vi "7-1.vi"() -> ()   [LabVIEW 2022 SP3, in "AoC22.lvlib"]
uses:
  AoC22.lvlib
  Disk Node.ctl
  <vilib>/IlluminatedG/lv-stream/Stream.lvlib
panel:
  out "Numeric":u64
  out "ABORT":bool
  in  "milliseconds to wait":u32
  out "elements":i32[](array[numeric])
  out "Array":T1[](array[typedef])
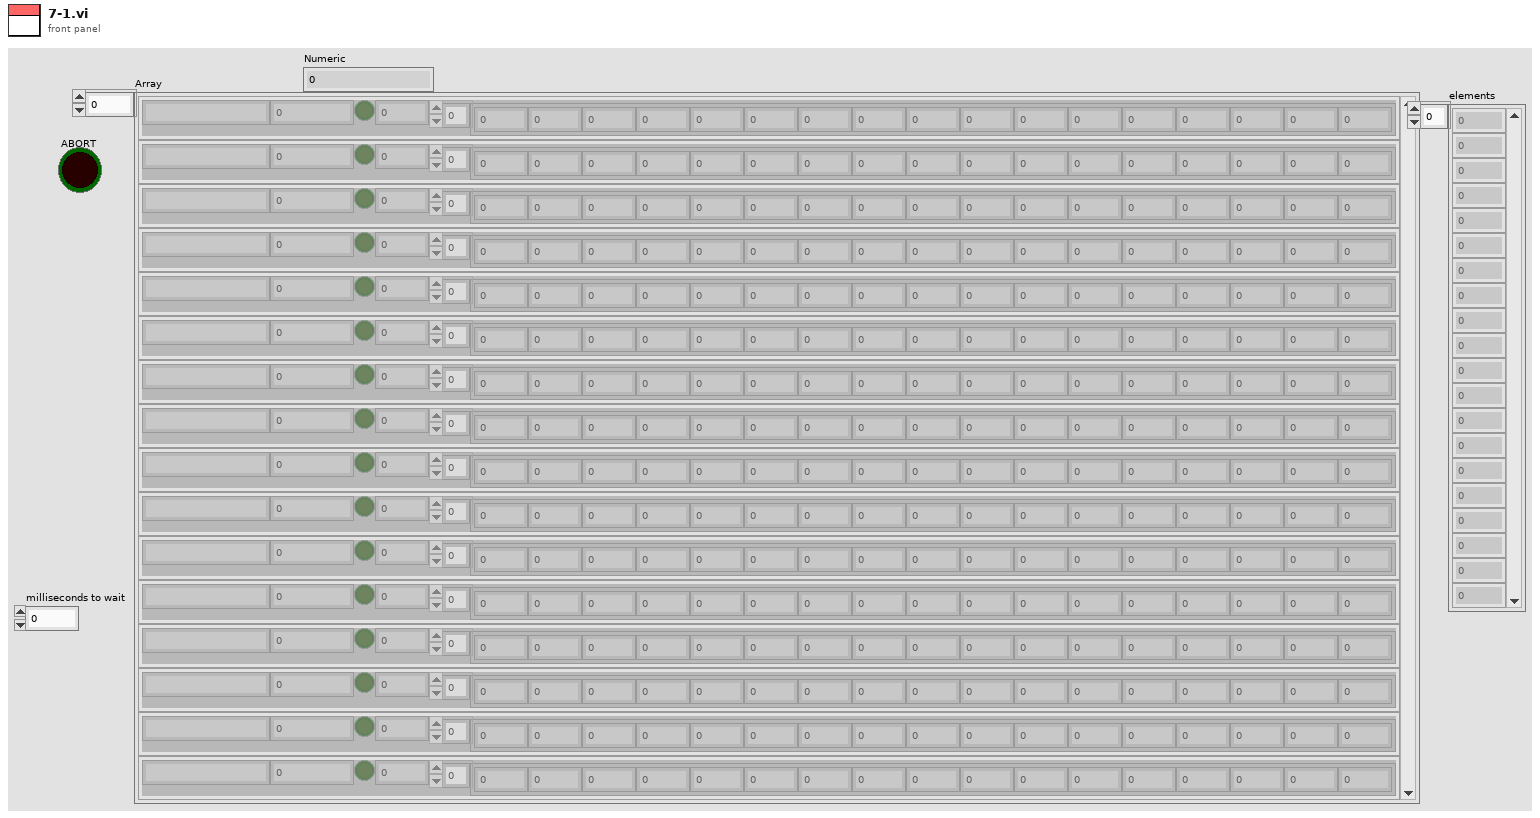
[diagram p1: front panel]
types:
  T1 = typedef "AoC22.lvlib/Disk Node.ctl" = cluster{"Name":string, "Size":u32, "Directory":bool, "Parent":i32, "Children":i32[]}
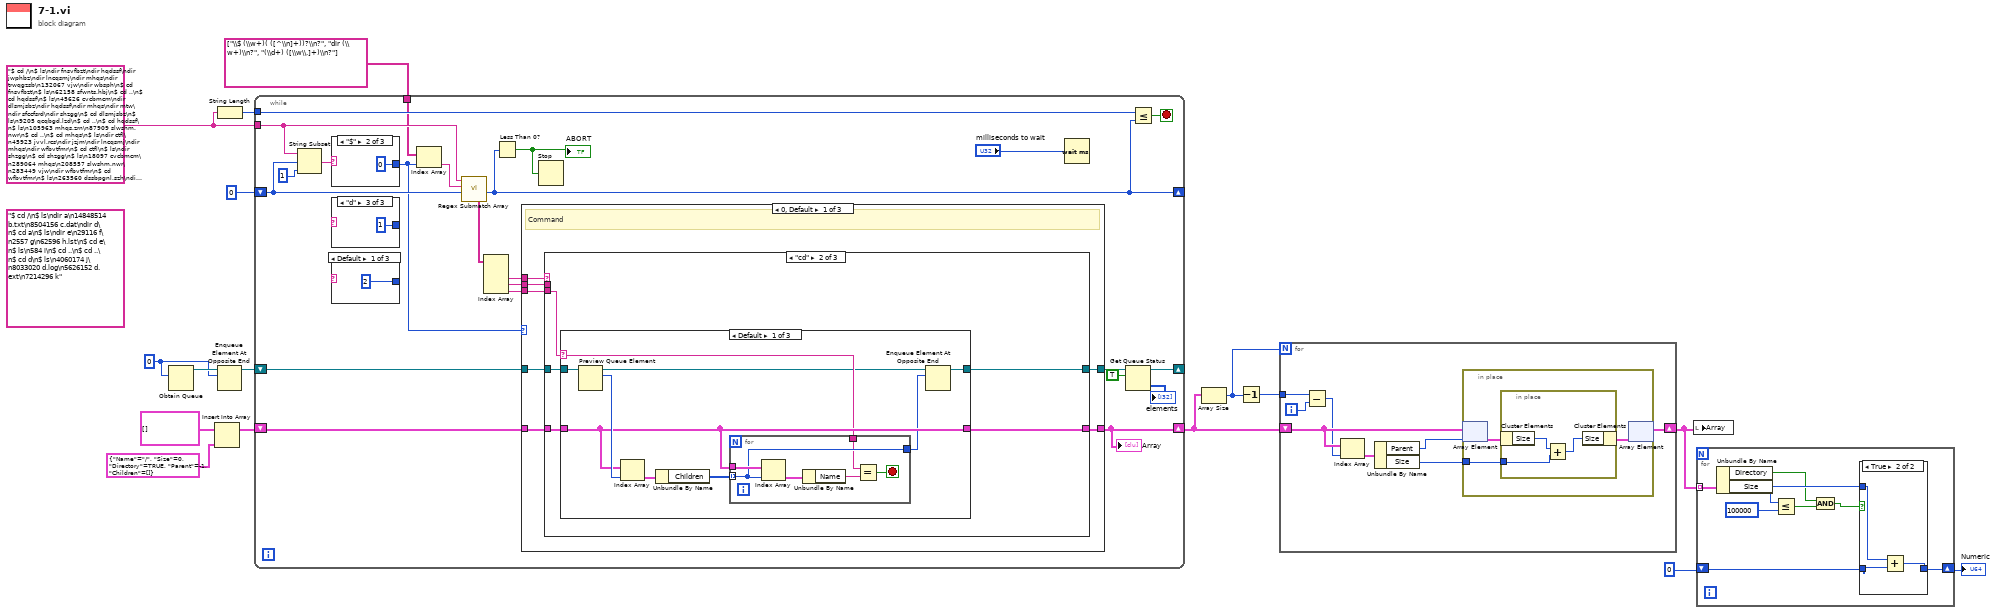
[diagram p0: block diagram]
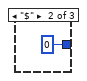
[diagram p3: hidden frame]
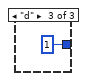
[diagram p4: hidden frame]
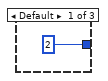
[diagram p5: hidden frame]
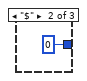
[diagram p6: hidden frame]
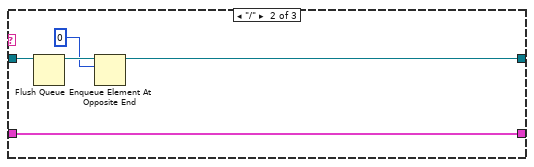
[diagram p8: hidden frame]
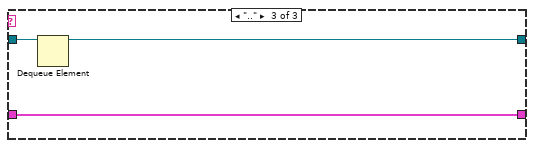
[diagram p9: hidden frame]
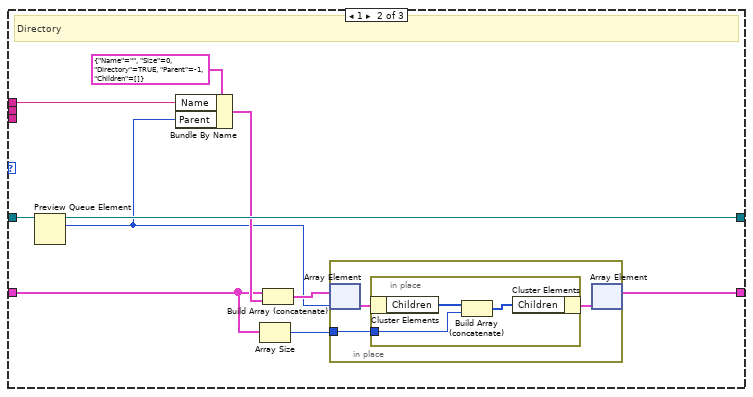
[diagram p11: hidden frame]
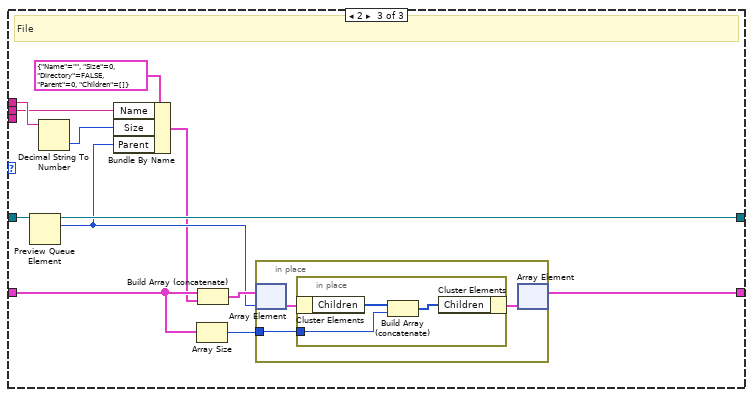
[diagram p12: hidden frame]
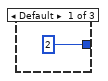
[diagram p13: hidden frame]
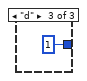
[diagram p14: hidden frame]
diagram:
  (unwired) "$ cd /\n$ ls\ndir a\n14848514 b.txt\n8504156 c.dat\ndir d\n$ cd a\n$ ls\ndir e\n29116 f\n2557 g\n62596 h.lst\n$ cd e\n$ ls\n584 i\n$ cd ..\n$ cd ..\n$ cd d\n$ ls\n4060174 j\n8033020 d.log\n5626152 d.ext\n7214296 k"
  w8 = 0
  w1 = "$ cd /\n$ ls\ndir fnsvfbzt\ndir hqdssf\ndir jwphbz\ndir lncqsmj\ndir mhqs\ndir trwqgzsb\n132067 vjw\ndir wbsph\n$ cd fnsvfbzt\n$ ls\n62158 sfwnts.hbj\n$ cd ..\n$ cd hqdssf\n$ ls\n45626 cvcbmcm\ndir dlsmjsbz\ndir hqdssf\ndir mhqs\ndir mtw\ndir sfccfsrd\ndir shzgg\n$ cd dlsmjsbz\n$ ls\n9205 qcqbgd.lzd\n$ cd ..\n$ cd hqdssf\n$ ls\n105963 mhqs.zrn\n87909 slwshm.nwr\n$ cd ..\n$ cd mhqs\n$ ls\ndir ctfl\n45923 jvvl.rcs\ndir jzjm\ndir lncqsmj\ndir mhqs\ndir wfbvtfmr\n$ cd ctfl\n$ ls\ndir shzgg\n$ cd shzgg\n$ ls\n18097 cvcbmcm\n289064 mhqs\n208557 slwshm.nwr\n283449 vjw\ndir wfbvtfmr\n$ cd wfbvtfmr\n$ ls\n263560 dssbpgnl.szh\ndir hnqjmq\n76551 jvvl.rcs\n195911 lncqsmj\n185776 slwshm.nwr\n$ cd hnqjmq\n$ ls\n3307 rjd.lgh\n$ cd ..\n$ cd ..\n$ cd ..\n$ cd ..\n$ cd jzjm\n$ ls\n31719 rjjrg.pjq\n$ cd ..\n$ cd lncqsmj\n$ ls\ndir mhqs\n$ cd mhqs\n$ ls\n138296 wfbvtfmr\n$ cd ..\n$ cd ..\n$ cd mhqs\n$ ls\n175499 jvvl.rcs\ndir rqznrr\n108476 slwshm.nwr\n199853 vjw\n$ cd rqznrr\n$ ls\n105075 shslmlt.spg\n$ cd ..\n$ cd ..\n$ cd wfbvtfmr\n$ ls\n131522 rjjrg.pjq\n$ cd ..\n$ cd ..\n$ cd mtw\n$ ls\ndir dcgpfrsf\ndir gwqm\n188911 hqdssf\n34693 jvvl.rcs\ndir shzgg\n$ cd dcgpfrsf\n$ ls\n47863 dfwthflp.jwq\n203815 dqbqbps.prq\ndir mhqs\n183653 rqjqpm.bbr\n220694 vjw\n$ cd mhqs\n$ ls\n74450 tjpn\n$ cd ..\n$ cd ..\n$ cd gwqm\n$ ls\ndir trghjhvs\n$ cd trghjhvs\n$ ls\ndir shzgg\n2620 slwshm.nwr\n$ cd shzgg\n$ ls\n73435 shzgg.bbf\n$ cd ..\n$ cd ..\n$ cd ..\n$ cd shzgg\n$ ls\n184378 rjjrg.pjq\n$ cd ..\n$ cd ..\n$ cd sfccfsrd\n$ ls\n87317 ccvs.phq\ndir cqmgf\ndir cssmfv\ndir hhhqdmz\n17971 mhqs\ndir mvjttqr\n264394 slwshm.nwr\ndir stdzptb\ndir tcddd\ndir zmrt\ndir zqqtb\n$ cd cqmgf\n$ ls\n202804 tcrqqlgs\n$ cd ..\n$ cd cssmfv\n$ ls\n13440 jnhzrtfd\n$ cd ..\n$ cd hhhqdmz\n$ ls\ndir fdbpld\n272827 jftd.lml\ndir prqbhbv\ndir wbzvmz\n$ cd fdbpld\n$ ls\ndir bgrnz\ndir dcdj\n78284 jqqfc.tzz\n147731 lbdsh.plp\n269235 ntf.gmq\n$ cd bgrnz\n$ ls\ndir qzs\ndir rcv\ndir wmrmhdd\n$ cd qzs\n$ ls\n156779 lncqsmj.gnf\n$ cd ..\n$ cd rcv\n$ ls\n224927 dvbw.svf\ndir hqdssf\ndir jjmsqft\n255189 mhqs.pcl\ndir mvgqtlm\ndir pjs\ndir sljw\n$ cd hqdssf\n$ ls\n63099 blpdwd\n96035 jvvl.rcs\n40533 lvpsmzw\n205031 rjjrg.pjq\n59874 shzgg.ldg\ndir zdnfpwlw\n$ cd zdnfpwlw\n$ ls\n109325 hqdssf.fmj\n41775 jfqhq.tdn\n203744 nprghch.zjb\ndir qfs\ndir rzctqrgm\ndir shzgg\n$ cd qfs\n$ ls\n234449 vjw\n$ cd ..\n$ cd rzctqrgm\n$ ls\n99041 cvcbmcm\n$ cd ..\n$ cd shzgg\n$ ls\n149752 mhqs.bds\n126331 rjjrg.pjq\n75464 vbcjqdjv\n$ cd ..\n$ cd ..\n$ cd ..\n$ cd jjmsqft\n$ ls\n47522 shzgg\n$ cd ..\n$ cd mvgqtlm\n$ ls\ndir tgtbj\ndir tmrsn\ndir vpv\n$ cd tgtbj\n$ ls\n86585 lbmv.jcr\n202755 rjjrg.pjq\n$ cd ..\n$ cd tmrsn\n$ ls\n150980 hqdssf.hmh\n$ cd ..\n$ cd vpv\n$ ls\n197783 jvvl.rcs\n$ cd ..\n$ cd ..\n$ cd pjs\n$ ls\n216539 cvcbmcm\n159509 jgfphj\n195297 pdgnb.qjd\n162974 rjjrg.pjq\n$ cd ..\n$ cd sljw\n$ ls\n61689 hqdssf.bbn\n$ cd ..\n$ cd ..\n$ cd wmrmhdd\n$ ls\n92888 msgcqfbf\n$ cd ..\n$ cd ..\n$ cd dcdj\n$ ls\n99280 mclcnw\n$ cd ..\n$ cd ..\n$ cd prqbhbv\n$ ls\n102589 bqlcds.pqp\n107625 mhqs\n281871 mvwvdtd.dzf\n$ cd ..\n$ cd wbzvmz\n$ ls\n287371 tnwgfw\n$ cd ..\n$ cd ..\n$ cd mvjttqr\n$ ls\ndir dtf\ndir frcqdb\ndir hqdssf\n55645 slwshm.nwr\ndir zdzchmtq\n$ cd dtf\n$ ls\n121764 cvcbmcm\n279094 lncqsmj\n68484 slwshm.nwr\n278387 vjw\n$ cd ..\n$ cd frcqdb\n$ ls\n233216 lncqsmj.mbd\n217901 slwshm.nwr\n$ cd ..\n$ cd hqdssf\n$ ls\ndir dgdtm\n260973 qnt\n231311 thdrddd.zmj\n160399 vjw\ndir vpqjmmf\n197241 vqvzsv.nzg\n$ cd dgdtm\n$ ls\ndir cnshbf\n173312 vjw\n$ cd cnshbf\n$ ls\n72788 hqdssf.mhc\n122945 rjjrg.pjq\n$ cd ..\n$ cd ..\n$ cd vpqjmmf\n$ ls\n127969 hqdssf.stc\n267724 lncqsmj\n55890 mhqs.mql\ndir tsbtz\n$ cd tsbtz\n$ ls\n244065 qqfnbd.nqv\n59649 qttbcgd.vtj\n$ cd ..\n$ cd ..\n$ cd ..\n$ cd zdzchmtq\n$ ls\n271886 lmphsmv\ndir nncghrr\n$ cd nncghrr\n$ ls\n180468 rjjrg.pjq\n$ cd ..\n$ cd ..\n$ cd ..\n$ cd stdzptb\n$ ls\n19398 frsztqqz.mnc\n$ cd ..\n$ cd tcddd\n$ ls\ndir hqdssf\n71084 jvvl.rcs\ndir wnzhld\n$ cd hqdssf\n$ ls\n178907 gcslqrn\n$ cd ..\n$ cd wnzhld\n$ ls\n206073 hpdnj\n$ cd ..\n$ cd ..\n$ cd zmrt\n$ ls\ndir bmfgjr\ndir bpztq\ndir chsh\ndir dpjhn\n288144 mhqs.zvb\n$ cd bmfgjr\n$ ls\n189592 jhmgm\n$ cd ..\n$ cd bpztq\n$ ls\n184906 rjjrg.pjq\n$ cd ..\n$ cd chsh\n$ ls\n110753 jvvl.rcs\ndir lncqsmj\ndir njdgplj\ndir qhpplfnd\n190460 rjjrg.pjq\n144668 wfbvtfmr.flv\n$ cd lncqsmj\n$ ls\ndir pzd\n$ cd pzd\n$ ls\n287833 vhfjdg.jrz\n$ cd ..\n$ cd ..\n$ cd njdgplj\n$ ls\ndir cbvz\ndir vfhj\n$ cd cbvz\n$ ls\ndir rtpcsrf\n$ cd rtpcsrf\n$ ls\n240018 wfbvtfmr\n$ cd ..\n$ cd ..\n$ cd vfhj\n$ ls\n152840 cbbrgc.wnq\n243656 hqdssf\n36325 hqdssf.fhn\n$ cd ..\n$ cd ..\n$ cd qhpplfnd\n$ ls\n206490 dfththnq.vnm\n$ cd ..\n$ cd ..\n$ cd dpjhn\n$ ls\n127322 rjjrg.pjq\ndir shzgg\n$ cd shzgg\n$ ls\n165774 cvcbmcm\n$ cd ..\n$ cd ..\n$ cd ..\n$ cd zqqtb\n$ ls\ndir ljnmbqvd\n60485 pcz.snl\n274930 slwshm.nwr\n131928 vqm\n51341 wfbvtfmr.stc\n$ cd ljnmbqvd\n$ ls\n268048 bdbjn\ndir fjh\ndir qpclpbz\ndir rqpljw\ndir tzjftf\n255809 vjw\n243604 wfbvtfmr.rzb\n$ cd fjh\n$ ls\n180021 hqdssf.rqs\n$ cd ..\n$ cd qpclpbz\n$ ls\n109952 blmm.nsv\ndir dltbt\ndir htbzp\n287761 mfbd\ndir mhqs\ndir vgbvrwvn\ndir wmhd\n$ cd dltbt\n$ ls\n205121 dfzlcv.hjf\n56409 hpqhhmb.sss\n233277 hqdssf.qcb\n187838 mbmcfhf.fnj\ndir rrqjn\ndir swrgj\n151306 tqjzq.dmg\n$ cd rrqjn\n$ ls\n240447 lncqsmj\n$ cd ..\n$ cd swrgj\n$ ls\ndir lnnwdbt\ndir sgjsn\ndir wfbvtfmr\n$ cd lnnwdbt\n$ ls\n213111 tnn.bhq\n$ cd ..\n$ cd sgjsn\n$ ls\ndir wpprqhs\n$ cd wpprqhs\n$ ls\ndir hqdssf\n$ cd hqdssf\n$ ls\n209286 qbdfzdzw.sgp\n$ cd ..\n$ cd ..\n$ cd ..\n$ cd wfbvtfmr\n$ ls\n199298 hqdssf.chs\n123953 rjjrg.pjq\n$ cd ..\n$ cd ..\n$ cd ..\n$ cd htbzp\n$ ls\ndir bmfr\n68162 bzwcswr.mlv\n284074 dtzwf\n270421 jpsvh.ncc\ndir mwbvz\n95631 shzgg.tbf\n44434 vjw\n$ cd bmfr\n$ ls\n19937 shzgg\n$ cd ..\n$ cd mwbvz\n$ ls\n156668 rjjrg.pjq\n$ cd ..\n$ cd ..\n$ cd mhqs\n$ ls\n111821 ftrv.zcw\ndir jsnlcn\ndir mhqs\ndir rjdwmb\ndir sfmrwgd\n$ cd jsnlcn\n$ ls\n7527 smqts.cnc\ndir svdw\n$ cd svdw\n$ ls\n173846 vjtrp\n$ cd ..\n$ cd ..\n$ cd mhqs\n$ ls\ndir hswdjgg\n30326 rjjrg.pjq\n$ cd hswdjgg\n$ ls\n285037 jvvl.rcs\n$ cd ..\n$ cd ..\n$ cd rjdwmb\n$ ls\n219498 twl.lmw\n$ cd ..\n$ cd sfmrwgd\n$ ls\n168290 ltwpm.fjl\n$ cd ..\n$ cd ..\n$ cd vgbvrwvn\n$ ls\ndir bswv\ndir hqdssf\ndir mhqs\n$ cd bswv\n$ ls\n121032 cncdt\ndir jrbmlg\ndir lncqsmj\ndir mhmgn\n65380 rjjrg.pjq\ndir wfbvtfmr\n$ cd jrbmlg\n$ ls\n37975 shzgg.bnq\n$ cd ..\n$ cd lncqsmj\n$ ls\n114558 jvvl.rcs\ndir mhqs\ndir nfn\ndir nhlbfq\n141816 phtt.phj\n181530 vjw\n224510 zmzp.jwg\n$ cd mhqs\n$ ls\ndir wpnw\n$ cd wpnw\n$ ls\n286077 lncqsmj.cld\n$ cd ..\n$ cd ..\n$ cd nfn\n$ ls\n269740 cvcbmcm\n87123 mhqs.nst\n61029 mhqs.vhb\n211712 slwshm.nwr\n$ cd ..\n$ cd nhlbfq\n$ ls\n247458 lncqsmj\n$ cd ..\n$ cd ..\n$ cd mhmgn\n$ ls\n85806 vjw\n$ cd ..\n$ cd wfbvtfmr\n$ ls\n275888 cvvhvg.pwv\n151703 gnbm\n61419 grcfbwdp\n150382 gzdmzj.wpc\ndir mtrqcwrd\n112827 nbtjlnt.srg\n$ cd mtrqcwrd\n$ ls\n273564 shzgg.tbm\n$ cd ..\n$ cd ..\n$ cd ..\n$ cd hqdssf\n$ ls\n72227 ccvwdrs.dsf\n141028 dctbz.spr\ndir shzgg\n277461 slwshm.nwr\n94390 stgp.trm\n24297 vgdzsrrl.dhg\n$ cd shzgg\n$ ls\n143437 lncqsmj.vpl\n78418 pbdwbmtd.nlp\n28173 vlfj.tps\n$ cd ..\n$ cd ..\n$ cd mhqs\n$ ls\n97312 jvvl.rcs\ndir qqfbsz\n42472 rjjrg.pjq\ndir wfbvtfmr\n$ cd qqfbsz\n$ ls\ndir lncqsmj\ndir mhqs\n$ cd lncqsmj\n$ ls\n186873 wfbvtfmr.lfh\n$ cd ..\n$ cd mhqs\n$ ls\ndir wfbvtfmr\n$ cd wfbvtfmr\n$ ls\n234441 gsjwsn\n$ cd ..\n$ cd ..\n$ cd ..\n$ cd wfbvtfmr\n$ ls\n55214 dgf\ndir fdtz\n6756 jvvl.rcs\n226995 rpsjvr.wpb\n68993 vjw\n$ cd fdtz\n$ ls\ndir rdzsjm\n$ cd rdzsjm\n$ ls\ndir mjgfpvc\n$ cd mjgfpvc\n$ ls\ndir vfcq\n$ cd vfcq\n$ ls\ndir fmtfm\n$ cd fmtfm\n$ ls\n200137 dvbqjq\n$ cd ..\n$ cd ..\n$ cd ..\n$ cd ..\n$ cd ..\n$ cd ..\n$ cd ..\n$ cd ..\n$ cd wmhd\n$ ls\ndir hnn\ndir rzt\n$ cd hnn\n$ ls\n16335 wfbvtfmr.vhw\n262909 zgtln.dwc\n$ cd ..\n$ cd rzt\n$ ls\n285086 mhqs.vsg\ndir qnr\n$ cd qnr\n$ ls\n290611 llnp.hsh\n$ cd ..\n$ cd ..\n$ cd ..\n$ cd ..\n$ cd rqpljw\n$ ls\n267152 jbv\n$ cd ..\n$ cd tzjftf\n$ ls\n258707 cnfb.dgv\n17087 hqdssf.dtd\n92075 nwvtww\ndir qblrnn\ndir tdg\n$ cd qblrnn\n$ ls\ndir brrqp\ndir frqcc\n25504 jvvl.rcs\ndir lncqsmj\ndir mhqs\n107908 rjjrg.pjq\n286918 rngbhp.ntg\ndir shzgg\ndir wcnh\ndir wfbvtfmr\n$ cd brrqp\n$ ls\n270783 wfbvtfmr\n$ cd ..\n$ cd frqcc\n$ ls\ndir clj\n7502 lncqsmj\ndir mnsbr\n73859 scwltjwh.cqd\n29920 vjw\ndir wpplgrc\n$ cd clj\n$ ls\n31407 grm.pwv\n$ cd ..\n$ cd mnsbr\n$ ls\ndir wfbvtfmr\n99467 whsrtf.gff\n$ cd wfbvtfmr\n$ ls\n81283 cvcbmcm\n$ cd ..\n$ cd ..\n$ cd wpplgrc\n$ ls\n285496 lncqsmj.hwq\n$ cd ..\n$ cd ..\n$ cd lncqsmj\n$ ls\n8972 jvvl.rcs\n$ cd ..\n$ cd mhqs\n$ ls\n119520 hqdssf.tbn\n$ cd ..\n$ cd shzgg\n$ ls\n180825 lncqsmj.rsg\n23507 wfbvtfmr\n$ cd ..\n$ cd wcnh\n$ ls\n98662 tmwrh\n220468 wml.sht\n$ cd ..\n$ cd wfbvtfmr\n$ ls\n283178 hqdssf.ctf\n$ cd ..\n$ cd ..\n$ cd tdg\n$ ls\n283636 cvcbmcm\n117742 gsqzjfn.pmp\n176660 lncqsmj\ndir pbdgbsts\ndir znvv\n$ cd pbdgbsts\n$ ls\n92092 vjw\n$ cd ..\n$ cd znvv\n$ ls\n41213 hqdssf.rnn\ndir pcttrtd\n$ cd pcttrtd\n$ ls\n16759 mhqs.gpb\n$ cd ..\n$ cd ..\n$ cd ..\n$ cd ..\n$ cd ..\n$ cd ..\n$ cd ..\n$ cd shzgg\n$ ls\n19544 bcn.rws\ndir fqwpwcq\ndir hngpzst\ndir hqdssf\ndir shzgg\ndir vgjr\ndir wfbvtfmr\n$ cd fqwpwcq\n$ ls\n269576 mhqs\ndir pmfv\n$ cd pmfv\n$ ls\n175725 jvvl.rcs\n29161 pnbm.mlr\n$ cd ..\n$ cd ..\n$ cd hngpzst\n$ ls\n18430 cvcbmcm\ndir fgzlgbm\ndir hqdssf\n378 rjjrg.pjq\ndir zjlnsztt\n$ cd fgzlgbm\n$ ls\n134751 dwlfbfjp\ndir hqdssf\n227313 jvvl.rcs\ndir lncqsmj\ndir mhqs\ndir qfjmtvpv\ndir qzm\n114934 shzgg.jdf\n187091 zpgbdnl.twq\n$ cd hqdssf\n$ ls\n87131 bdmdpdf.cqg\ndir fdc\ndir gwgp\n$ cd fdc\n$ ls\n116738 cvcbmcm\n$ cd ..\n$ cd gwgp\n$ ls\ndir qdvss\ndir rpwzw\ndir wfbvtfmr\n$ cd qdvss\n$ ls\n111546 wqnsrnh\n$ cd ..\n$ cd rpwzw\n$ ls\n183614 lfjqvff\n129803 rdwd\n$ cd ..\n$ cd wfbvtfmr\n$ ls\n266779 mhqs\n189793 slwshm.nwr\n279894 sncqtvwp.mff\n40520 vjw\n$ cd ..\n$ cd ..\n$ cd ..\n$ cd lncqsmj\n$ ls\n257714 dtcjv.lsd\n69877 shzgg\n267645 vjw\n$ cd ..\n$ cd mhqs\n$ ls\n257031 stsfrb.gvs\n$ cd ..\n$ cd qfjmtvpv\n$ ls\ndir mhqs\n$ cd mhqs\n$ ls\n91378 wldhvhl\n$ cd ..\n$ cd ..\n$ cd qzm\n$ ls\ndir shn\n$ cd shn\n$ ls\ndir jmmlsvdg\n$ cd jmmlsvdg\n$ ls\n41383 rnlgl.vjv\n$ cd ..\n$ cd ..\n$ cd ..\n$ cd ..\n$ cd hqdssf\n$ ls\ndir mzj\n$ cd mzj\n$ ls\n169639 sgdn\n$ cd ..\n$ cd ..\n$ cd zjlnsztt\n$ ls\n78315 jfj.sgg\n$ cd ..\n$ cd ..\n$ cd hqdssf\n$ ls\n906 rjjrg.pjq\n$ cd ..\n$ cd shzgg\n$ ls\n163015 mhqs.cnb\n$ cd ..\n$ cd vgjr\n$ ls\n129546 hclg.vbl\n286437 hqdssf\ndir lncqsmj\n1552 nhgwff\n279693 qmpdlw\n83645 slwshm.nwr\n$ cd lncqsmj\n$ ls\n233355 fhpjbpjl.tbh\n$ cd ..\n$ cd ..\n$ cd wfbvtfmr\n$ ls\n218452 jvvl.rcs\n47525 rjjrg.pjq\n109880 tctz.rnd\n$ cd ..\n$ cd ..\n$ cd ..\n$ cd jwphbz\n$ ls\ndir bqbwds\ndir mwnzw\n113414 qgdsgfg.ngj\n141013 qtp\n10795 slwshm.nwr\n$ cd bqbwds\n$ ls\n18049 shzgg\n$ cd ..\n$ cd mwnzw\n$ ls\n169353 dtqlr\ndir hlrgzlph\ndir mhqs\n238527 vjw\n$ cd hlrgzlph\n$ ls\n249097 hqdssf\n86490 pwdmzwb\n$ cd ..\n$ cd mhqs\n$ ls\n176337 rjjrg.pjq\n$ cd ..\n$ cd ..\n$ cd ..\n$ cd lncqsmj\n$ ls\ndir jmsw\ndir mcgm\ndir mpc\n233050 rjjrg.pjq\n30757 shzgg\n250575 slwshm.nwr\n$ cd jmsw\n$ ls\ndir hqdssf\ndir nmsbdqhm\ndir wfbvtfmr\n$ cd hqdssf\n$ ls\n44806 lvzm\n$ cd ..\n$ cd nmsbdqhm\n$ ls\ndir czzp\ndir gcp\ndir gsrnmq\ndir rmngvc\ndir vpfq\ndir vpzvb\ndir wccgblsq\n43981 wfbvtfmr\n$ cd czzp\n$ ls\n95330 slwshm.nwr\n82000 wfbvtfmr\n$ cd ..\n$ cd gcp\n$ ls\n229303 ddsppspd.fcn\n$ cd ..\n$ cd gsrnmq\n$ ls\ndir hrsstlt\ndir rzc\n40890 sfpt\n$ cd hrsstlt\n$ ls\n18477 mnpc.tmh\n$ cd ..\n$ cd rzc\n$ ls\n33078 dmfwf\n149792 wfbvtfmr.jnz\ndir zsnmz\n$ cd zsnmz\n$ ls\ndir gzsnl\n69834 lplszs.rvg\n213489 slwshm.nwr\ndir vrnqh\n$ cd gzsnl\n$ ls\n109060 jvvl.rcs\n122307 svtppnvt.wrz\n$ cd ..\n$ cd vrnqh\n$ ls\n94389 jvvl.rcs\n$ cd ..\n$ cd ..\n$ cd ..\n$ cd ..\n$ cd rmngvc\n$ ls\ndir jljbrrgg\n$ cd jljbrrgg\n$ ls\n128554 cvcbmcm\n$ cd ..\n$ cd ..\n$ cd vpfq\n$ ls\n73628 rjjrg.pjq\n$ cd ..\n$ cd vpzvb\n$ ls\n265609 rjjrg.pjq\n$ cd ..\n$ cd wccgblsq\n$ ls\n110134 hffzwm.zfr\n$ cd ..\n$ cd ..\n$ cd wfbvtfmr\n$ ls\n209356 jvvl.rcs\n286105 mtsb.bwd\n234687 vcgnlc.cft\n$ cd ..\n$ cd ..\n$ cd mcgm\n$ ls\n203407 cvcbmcm\n$ cd ..\n$ cd mpc\n$ ls\ndir shzgg\n$ cd shzgg\n$ ls\ndir bnb\n$ cd bnb\n$ ls\n232449 lncqsmj.czs\n$ cd ..\n$ cd ..\n$ cd ..\n$ cd ..\n$ cd mhqs\n$ ls\n116955 jvvl.rcs\n$ cd ..\n$ cd trwqgzsb\n$ ls\n88439 jgphdrnq\n$ cd ..\n$ cd wbsph\n$ ls\ndir mhqs\ndir vgh\n$ cd mhqs\n$ ls\n133965 rfh.zdb\n$ cd ..\n$ cd vgh\n$ ls\n36092 rjjrg.pjq"
  n1 = Obtain Queue(element data type=w8) -> (queue out=w10:refnum<queue>)  [unwired: 4 in, 2 out]
  n2 = Insert Into Array(array=T1[] [], new element=T1 {"Name"="/", "Size"=0, "Directory"=TRUE, "Parent"=-1, "Children"=[]} ("new element/subarray")) -> (w12:T1[])  [unwired: 1 in]
  n3 = Enqueue Element At Opposite End(queue=w10, element=w8) -> (queue out=w9:refnum<queue>)  [unwired: 2 in, 2 out]
  n4 = String Length(string=w1) -> (length=w15:i32)
  n5 = while {
    tunnel: w1 -> [w36]
    shift-right: [w26] -> _
    shift-left: 0 -> [w35]
    tunnel: w15 -> [w39]
    shift-right: [w24] -> _
    shift-left: w9 -> [w18]
    shift-right: [w19] -> w7
    shift-left: w12 -> [w17]
    tunnel: string[] ["\\$ (\\w+)( ([^\\n]+))?\\n?", "dir (\\w+)\\n?", "(\\d+) ([\\w\\.]+)\\n?"] -> [w32]
    stop <- w38 stop-if-true
    n6 = String Subset(string=w36, offset (0)=w35, length (rest)=1 ("length (rest)")) -> (substring=w33:string)
    n7 = case shown="\"$\"" w33 {
      tunnel: [2 0 1] -> w30
      frame Default {
      }
      frame "$" {
      }
      frame "d" {
      }
    }
    n8 = case shown="\"d\"" {
      selector: _ -> [_ _ _]
      tunnel: [2 0 1] -> _
      frame Default {
      }
      frame "$" {
      }
      frame "d" {
      }
    }
    n9 = case shown="Default" {
      selector: _ -> [_ _ _]
      tunnel: [2 0 1] -> _
      frame Default {
      }
      frame "$" {
      }
      frame "d" {
      }
    }
    n10 = Index Array(array=w32, index=w30) -> (element=w31:string)
    n11 = call <vilib>:"Regex Submatch Array.vi"("offset (0)"=w35, "regular expression"=w31, "string"=w36) -> ("offset past match"=w26:i32, "matches"=w37:string[])  [unwired: 6 in, 1 out]
    n12 = Index Array(array=w37) -> (element #2=w29:string, element #3=w28:string, element #4=w20:string)  [unwired: 4 in, 1 out]
    n13 = Less Than 0?(x=w26) -> (x < 0?=w25:bool)
    "ABORT" <- w25
    n14 = case shown="0, Default" w30 {
      tunnel: w29 -> [w52 w91 w112]
      tunnel: w28 -> [w47 _ w111]
      tunnel: w18 -> [w51 w94 w109]
      tunnel: w17 -> [w49 w89 w107]
      tunnel: [w50 w93 w108] -> w27
      tunnel: [w48 w85 w103] -> w19
      tunnel: w20 -> [w46 _ _]
      frame 0, Default {
        # "Command"
        n15 = case shown="\"cd\"" w52 {
          tunnel: w51 -> [w54 w59 w84]
          tunnel: [w54 w57 w84] -> w50
          tunnel: w49 -> [w53 w58 w83]
          tunnel: [w53 w56 w83] -> w48
          tunnel: w47 -> [_ _ _]
          tunnel: w46 -> [_ w55 _]
          frame Default {
          }
          frame "cd" {
            n16 = case shown="Default" w55 {
              selector: w55 -> [w63 _ _]
              tunnel: w59 -> [w68 w79 w82]
              tunnel: w58 -> [w64 w78 w80]
              tunnel: [w61 w76 w81] -> w57
              tunnel: [w64 w78 w80] -> w56
              frame Default {
                n17 = Preview Queue Element(queue=w68) -> (queue out=w62:refnum<queue>, element=w67:i32)  [unwired: 2 in, 2 out]
                n18 = Index Array(array=w64, index=w67) -> (element=w66:T1)
                n19 = Unbundle By Name(w66) -> ("Children"=w65:i32[])
                n20 = for {
                  tunnel: w64 -> [w74]
                  tunnel: w65 -> [w72] mode=indexing
                  tunnel: [w72] -> w60
                  tunnel: w63 -> [w70]
                  stop <- w69 stop-if-true
                  n21 = Index Array(array=w74, index=w72) -> (element=w73:T1)
                  n22 = Unbundle By Name(w73) -> ("Name"=w71:string)
                  n23 = Equal?(x=w70, y=w71) -> (x = y?=w69:bool)
                }
                n24 = Enqueue Element At Opposite End(queue=w62, element=w60) -> (queue out=w61:refnum<queue>)  [unwired: 2 in, 2 out]
              }
              frame "/" {
                n25 = Flush Queue(queue=w79) -> (queue out=w77:refnum<queue>)  [unwired: 1 in, 2 out]
                n26 = Enqueue Element At Opposite End(queue=w77, element=0) -> (queue out=w76:refnum<queue>)  [unwired: 2 in, 2 out]
              }
              frame ".." {
                n27 = Dequeue Element(queue=w82) -> (queue out=w81:refnum<queue>)  [unwired: 2 in, 3 out]
              }
            }
          }
          frame "ls" {
          }
        }
      }
      frame 1 {
        # "Directory"
        n28 = Preview Queue Element(queue=w94) -> (queue out=w93:refnum<queue>, element=w86:i32)  [unwired: 2 in, 2 out]
        n29 = Bundle By Name(cluster=T1 {"Name"="", "Size"=0, "Directory"=TRUE, "Parent"=-1, "Children"=[]} ("new element/subarray"), "Name"=w91, "Parent"=w86) -> (w90:T1)
        n30 = Array Size(array=w89) -> (size(s)=w87:i32)
        n31 = Build Array (concatenate)(w89, w90) -> (w88:T1[])
        n32 = in-place {
          in-place-border: w87 -> [w96]
          n33 = in-place-array #1(w88, w86) -> (w97:T1)
          n34 = in-place {
            in-place-border: w96 -> [w99]
            n35 = in-place-cluster #2(w97) -> ("Children"=w100:i32[])
            n36 = Build Array (concatenate)(w100, w99) -> (w98:i32[])
            n37 = in-place-cluster #2("Children"=w98) -> (w95:T1)
          }
          n38 = in-place-array #1(w95) -> (w85:T1[])  [unwired: 1 out]
        }
      }
      frame 2 {
        # "File"
        n39 = Preview Queue Element(queue=w109) -> (queue out=w108:refnum<queue>, element=w102:i32)  [unwired: 2 in, 2 out]
        n40 = Decimal String To Number(string=w112) -> (number=w110:i32)  [unwired: 2 in, 1 out]
        n41 = Bundle By Name(cluster=T1 {"Name"="", "Size"=0, "Directory"=FALSE, "Parent"=0, "Children"=[]} ("new element/subarray"), "Name"=w111, "Size"=w110, "Parent"=w102) -> (w101:T1)
        n42 = Array Size(array=w107) -> (size(s)=w104:i32)
        n43 = Build Array (concatenate)(w107, w101) -> (w105:T1[])
        n44 = in-place {
          in-place-border: w104 -> [w114]
          n45 = in-place-array #3(w105, w102) -> (w115:T1)
          n46 = in-place {
            in-place-border: w114 -> [w117]
            n47 = in-place-cluster #4(w115) -> ("Children"=w118:i32[])
            n48 = Build Array (concatenate)(w118, w117) -> (w116:i32[])
            n49 = in-place-cluster #4("Children"=w116) -> (w113:T1)
          }
          n50 = in-place-array #3(w113) -> (w103:T1[])  [unwired: 1 out]
        }
      }
    }
    "Array" <- w19
    n51 = Stop(stop? (T)=w25) -> ()
    n52 = Wait (ms)(milliseconds to wait="milliseconds to wait") -> ()  [unwired: 1 out]
    n53 = Get Queue Status(queue=w27, return elements? (F)=TRUE) -> (queue out=w24:refnum<queue>, elements=→"elements":i32[])  [unwired: 1 in, 6 out]
    n54 = Less Or Equal?(x=w39, y=w26) -> (x <= y?=w38:bool)
  }
  n55 = Array Size(array=w7) -> (size(s)=w6:i32)
  n56 = Decrement(x=w6) -> (x-1=w5:i32)
  n57 = for {
    N: w6 -> [_]
    shift-right: [w127] -> w3
    shift-left: w7 -> [w126]
    tunnel: w5 -> [w129]
    i -> [w128]
    n58 = Subtract(x=w129, y=w128) -> (x-y=w125:i32)
    n59 = Index Array(array=w126, index=w125) -> (element=w124:T1)
    n60 = Unbundle By Name(w124) -> ("Parent"=w123:i32, "Size"=w122:u32)
    n61 = in-place {
      in-place-border: w122 -> [w130]
      n62 = in-place-array #5(w126, w123) -> (w132:T1)
      n63 = in-place {
        in-place-border: w130 -> [w133]
        n64 = in-place-cluster #6(w132) -> ("Size"=w135:u32)
        n65 = Add(x=w135, y=w133) -> (x+y=w134:u32)
        n66 = in-place-cluster #6("Size"=w134) -> (w131:T1)
      }
      n67 = in-place-array #5(w131) -> (w127:T1[])  [unwired: 1 out]
    }
  }
  n68 = local write "Array"(w3) -> ()
  n69 = for {
    shift-right: [w138] -> w2
    shift-left: u64 0 -> [w139]
    tunnel: w3 -> [w143] mode=indexing
    n70 = Unbundle By Name(w143) -> ("Directory"=w136:bool, "Size"=w140:u32)
    n71 = Less Or Equal?(x=w140, y=u32 100000) -> (x <= y?=w141:bool)
    n72 = And(x=w136, y=w141) -> (x .and. y?=w137:bool)
    n73 = case shown="True" w137 {
      tunnel: w140 -> [_ w146]
      tunnel: w139 -> [w144 w147]
      tunnel: [w144 w145] -> w138
      frame False {
      }
      frame True {
        n74 = Add(x=w146, y=w147) -> (x+y=w145:u64)
      }
    }
  }
  "Numeric" <- w2
